vi "SM Polling - Leave State if FALSE.vi"(11 "Boolean Condition":bool) -> (3 "Polling Action":T1)   [LabVIEW 2020, in "StateMachine.lvlib" / "HSE-State-Machine.lvlib"]
doc: "<b>Keep polling</b> if the boolean condition is TRUE\n____\nHAMPEL SOFTWARE ENGINEERING v2.6.0 (2023-12-19 10:54)"
uses:
  HSE-State-Machine.lvlib
  SM Polling Actions--enum.ctl
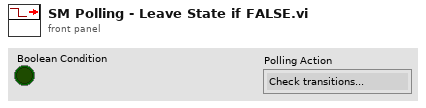
[diagram p1: front panel]
types:
  T1 = typedef "StateMachine.lvlib/HSE-State-Machine.lvlib/SM Polling Actions--enum.ctl" = enum16{"Check transitions...", "Leave this state!"}
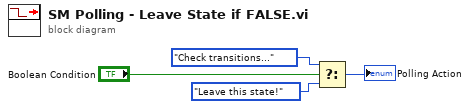
[diagram p0: block diagram]
diagram:
  n1 = Select(t=SM_Polling_Actions--enum."Check transitions..." ("SM Polling Actions"), s="Boolean Condition", f=SM_Polling_Actions--enum."Leave this state!" ("SM Polling Actions")) -> (s? t:f=→"Polling Action":T1)
